vi "toml_parse_string.vi"(8 "error in (no error)":errorcluster, 10 "allow_multiline? (T)":bool=TRUE, 11 "string":string) -> (0 "error out":errorcluster, 2 "value":variant, 3 "remaining string":string)   [LabVIEW 2017]
uses:
  <vilib>/Utility/error.llb/Error Cluster From Error Code.vi
  <vilib>/regexp/Match Regular Expression.xnode
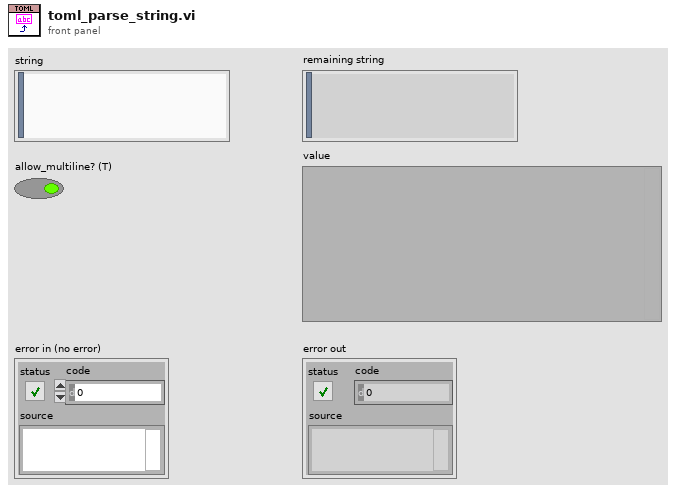
[diagram p1: front panel]
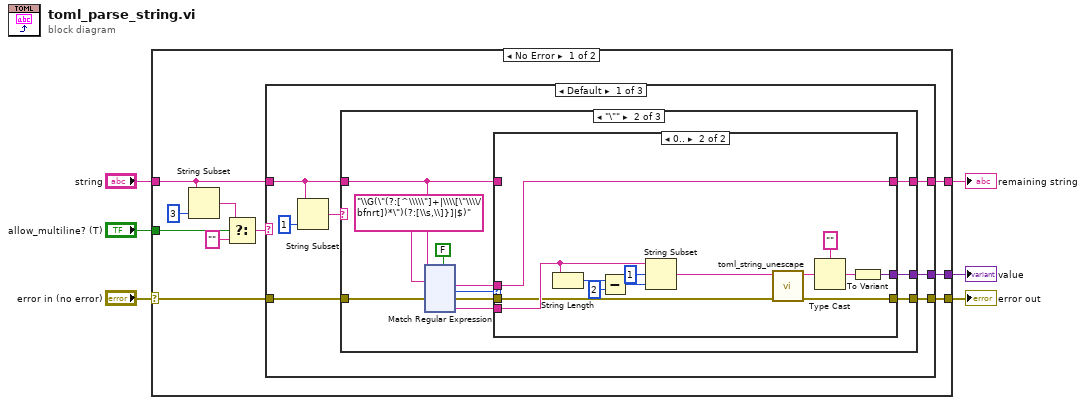
[diagram p0: block diagram]
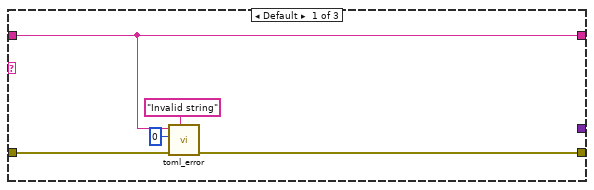
[diagram p2: hidden frame]
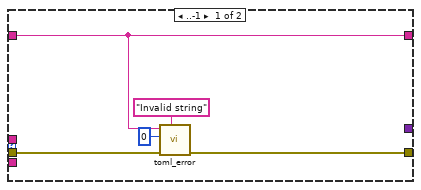
[diagram p3: hidden frame]
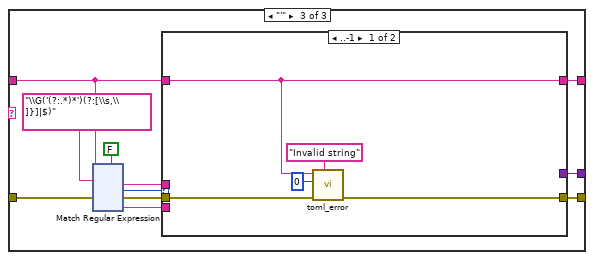
[diagram p4: hidden frame]
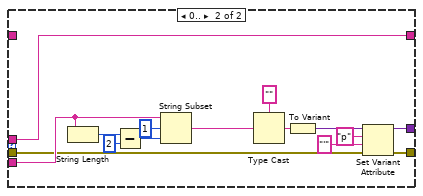
[diagram p5: hidden frame]
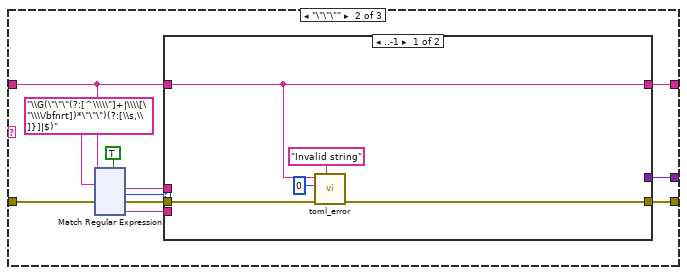
[diagram p6: hidden frame]
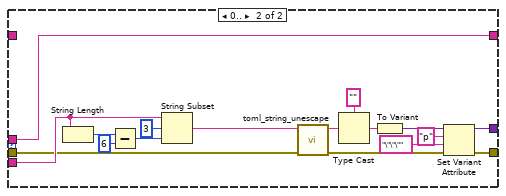
[diagram p7: hidden frame]
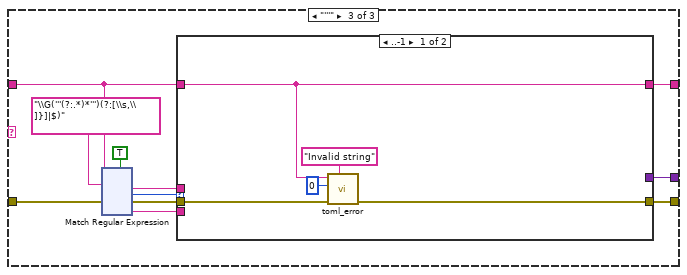
[diagram p8: hidden frame]
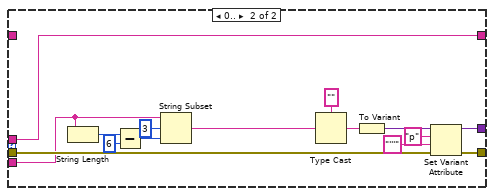
[diagram p9: hidden frame]
diagram:
  n1 = case shown="No Error" "error in (no error)" {
    selector: "error in (no error)" -> [w16 w616]
    tunnel: "string" -> [w15 w615]
    tunnel: [w13 w616] -> w4
    tunnel: [w12 w615] -> w3
    tunnel: [w11 _] -> w2
    tunnel: "allow_multiline? (T)" -> [w10 _]
    frame No Error {
      n2 = String Subset(string=w15, length (rest)=3 ("length (rest)")) -> (substring=w8:string)  [unwired: 1 in]
      n3 = Select(t=w8, s=w10, f="") -> (s? t:f=w7:string)
      n4 = case shown="Default" w7 {
        tunnel: w16 -> [w23 w329 w477]
        tunnel: w15 -> [w17 w324 w472]
        tunnel: [w22 w327 w475] -> w13
        tunnel: [w21 w325 w473] -> w12
        tunnel: [w20 w322 w470] -> w11
        frame Default {
          n5 = String Subset(string=w17, length (rest)=1 ("length (rest)")) -> (substring=w18:string)  [unwired: 1 in]
          n6 = case shown="\"\\\"\"" w18 {
            tunnel: w23 -> [w26 w38 w182]
            tunnel: [w25 w36 w180] -> w22
            tunnel: [w24 w34 w178] -> w21
            tunnel: w17 -> [w24 w33 w177]
            tunnel: [_ w31 w175] -> w20
            frame Default {
              n7 = call "toml_error.vi"("message"="Invalid string", "error in (no error)"=w26, "offset (0)"=0, "toml"=w24) -> ("error out"=w25:errorcluster)  [unwired: 7 in]
            }
            frame "\"" {
              n8 = xnode "Match Regular Expression"("input string"=w33, "regular expression"="\\G(\"(?:[^\\\\\"]+|\\\\[\"\\\\/bfnrt])*\")(?:[\\s,\\]}]|$)", "error in"=w38, "multiline? (F)"=FALSE) -> ("after match"=w32:string, "offset past match"=w37:i32, "error out"=w35:errorcluster, "submatch 1"=w29:string)  [unwired: 2 in, 2 out]
              n9 = case shown="0.." w37 {
                tunnel: [w43 w45] -> w36
                tunnel: w35 -> [w44 w45]
                tunnel: [w42 w56] -> w34
                tunnel: w33 -> [w42 _]
                tunnel: w32 -> [_ w56]
                tunnel: [_ w46] -> w31
                tunnel: w29 -> [_ w55]
                frame ..-1 {
                  n10 = call "toml_error.vi"("message"="Invalid string", "error in (no error)"=w44, "offset (0)"=0, "toml"=w42) -> ("error out"=w43:errorcluster)  [unwired: 7 in]
                }
                frame 0.. {
                  n11 = String Length(string=w55) -> (length=w51:i32)
                  n12 = Subtract(x=w51, y=2 ("x")) -> (x-y=w50:i32)
                  n13 = String Subset(string=w55, offset (0)=1, length (rest)=w50) -> (substring=w53:string)
                  n14 = call "toml_string_unescape.vi"("escaped string"=w53) -> ("string out"=w52:string)  [unwired: 9 in, 1 out]
                  n15 = Type Cast(type="", x=w52) -> (*(type *) &x=w48:string)
                  n16 = To Variant(anything=w48) -> (Variant=w46:variant)
                }
              }
            }
            frame "'" {
              n17 = xnode "Match Regular Expression"("input string"=w177, "regular expression"="\\G('(?:.*)*')(?:[\\s,\\]}]|$)", "error in"=w182, "multiline? (F)"=FALSE) -> ("after match"=w176:string, "offset past match"=w181:i32, "error out"=w179:errorcluster, "submatch 1"=w173:string)  [unwired: 2 in, 2 out]
              n18 = case shown="..-1" w181 {
                tunnel: [w187 w191] -> w180
                tunnel: w179 -> [w188 w192]
                tunnel: [w186 w203] -> w178
                tunnel: w177 -> [w186 _]
                tunnel: w176 -> [_ w203]
                tunnel: [_ w190] -> w175
                tunnel: w173 -> [_ w202]
                frame ..-1 {
                  n19 = call "toml_error.vi"("message"="Invalid string", "error in (no error)"=w188, "offset (0)"=0, "toml"=w186) -> ("error out"=w187:errorcluster)  [unwired: 7 in]
                }
                frame 0.. {
                  n20 = String Length(string=w202) -> (length=w200:i32)
                  n21 = Subtract(x=w200, y=2 ("x")) -> (x-y=w199:i32)
                  n22 = String Subset(string=w202, offset (0)=1, length (rest)=w199) -> (substring=w197:string)
                  n23 = Type Cast(type="", x=w197) -> (*(type *) &x=w196:string)
                  n24 = To Variant(anything=w196) -> (Variant=w189:variant)
                  n25 = Set Variant Attribute(Variant=w189, name="p", value="'", error in=w192) -> (Variant out=w190:variant, error out=w191:errorcluster)  [unwired: 1 out]
                }
              }
            }
          }
        }
        frame "\"\"\"" {
          n26 = xnode "Match Regular Expression"("input string"=w324, "regular expression"="\\G(\"\"\"(?:[^\\\\\"]+|\\\\[\"\\\\/bfnrt])*\"\"\")(?:[\\s,\\]}]|$)", "error in"=w329, "multiline? (F)"=TRUE) -> ("after match"=w323:string, "offset past match"=w328:i32, "error out"=w326:errorcluster, "submatch 1"=w320:string)  [unwired: 2 in, 2 out]
          n27 = case shown="..-1" w328 {
            tunnel: [w334 w340] -> w327
            tunnel: w326 -> [w335 w341]
            tunnel: [w333 w351] -> w325
            tunnel: w324 -> [w333 _]
            tunnel: w323 -> [_ w351]
            tunnel: [_ w338] -> w322
            tunnel: w320 -> [_ w350]
            frame ..-1 {
              n28 = call "toml_error.vi"("message"="Invalid string", "error in (no error)"=w335, "offset (0)"=0, "toml"=w333) -> ("error out"=w334:errorcluster)  [unwired: 7 in]
            }
            frame 0.. {
              n29 = String Length(string=w350) -> (length=w346:i32)
              n30 = Subtract(x=w346, y=6 ("x")) -> (x-y=w345:i32)
              n31 = String Subset(string=w350, offset (0)=3, length (rest)=w345) -> (substring=w348:string)
              n32 = call "toml_string_unescape.vi"("escaped string"=w348) -> ("string out"=w347:string)  [unwired: 9 in, 1 out]
              n33 = Type Cast(type="", x=w347) -> (*(type *) &x=w343:string)
              n34 = To Variant(anything=w343) -> (Variant=w339:variant)
              n35 = Set Variant Attribute(Variant=w339, name="p", value="\"\"\"", error in=w341) -> (Variant out=w338:variant, error out=w340:errorcluster)  [unwired: 1 out]
            }
          }
        }
        frame "'''" {
          n36 = xnode "Match Regular Expression"("input string"=w472, "regular expression"="\\G('''(?:.*)*''')(?:[\\s,\\]}]|$)", "error in"=w477, "multiline? (F)"=TRUE) -> ("after match"=w471:string, "offset past match"=w476:i32, "error out"=w474:errorcluster, "submatch 1"=w468:string)  [unwired: 2 in, 2 out]
          n37 = case shown="..-1" w476 {
            tunnel: [w482 w488] -> w475
            tunnel: w474 -> [w483 w497]
            tunnel: [w481 w498] -> w473
            tunnel: w472 -> [w481 _]
            tunnel: w471 -> [_ w498]
            tunnel: [_ w486] -> w470
            tunnel: w468 -> [_ w496]
            frame ..-1 {
              n38 = call "toml_error.vi"("message"="Invalid string", "error in (no error)"=w483, "offset (0)"=0, "toml"=w481) -> ("error out"=w482:errorcluster)  [unwired: 7 in]
            }
            frame 0.. {
              n39 = String Length(string=w496) -> (length=w494:i32)
              n40 = Subtract(x=w494, y=6 ("x")) -> (x-y=w493:i32)
              n41 = String Subset(string=w496, offset (0)=3, length (rest)=w493) -> (substring=w491:string)
              n42 = Type Cast(type="", x=w491) -> (*(type *) &x=w490:string)
              n43 = To Variant(anything=w490) -> (Variant=w487:variant)
              n44 = Set Variant Attribute(Variant=w487, name="p", value="'''", error in=w497) -> (Variant out=w486:variant, error out=w488:errorcluster)  [unwired: 1 out]
            }
          }
        }
      }
    }
    frame Error {
    }
  }
  "error out" <- w4
  "remaining string" <- w3
  "value" <- w2
